vi "Dialog Window YN.vi"(6 "Front Panel Window:Panel Bounds":T2, 7 "Üzenet be":string, 8 "Error In":errorcluster, 10 "Message":T1, 11 "Message Queue":refnum<queue>) -> (0 "Error Out":errorcluster)   [LabVIEW 2014]
uses:
  <vilib>/Utility/miscctls.llb/LVRectTypeDef.ctl
  Message.ctl
  support/Message Queue/Message Cluster.ctl
  Teszt/Teszt.ctl
  Teszt/Command.ctl
  support/Message Queue/Enqueue Message (Single).vi
  support/Message Queue/Message Queue.lvlib
panel:
  in  "Nem":bool
  out "Üzenet":string
  in  "Igen":bool
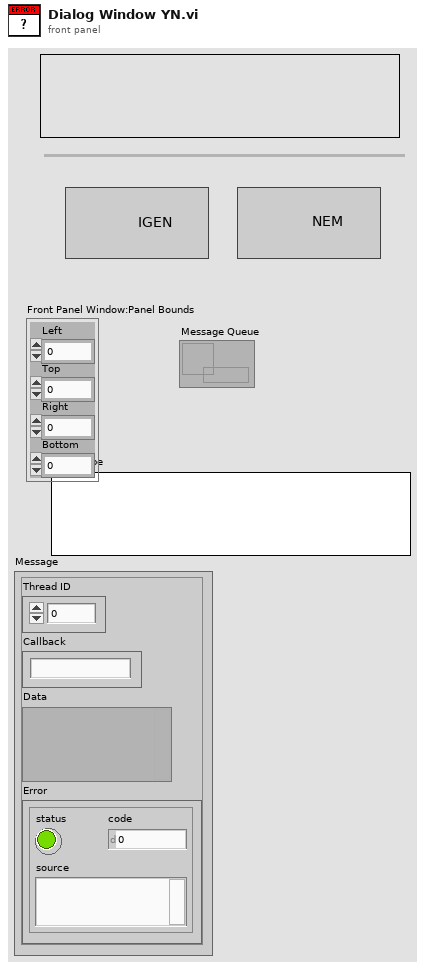
[diagram p1: front panel]
types:
  T1 = typedef "Message.ctl" = cluster{"Thread ID":u16, "Callback":string, "Data":variant, "Error":errorcluster}
  T2 = typedef "LVRectTypeDef.ctl" = cluster{"Left":i16, "Top":i16, "Right":i16, "Bottom":i16}
  T3 = typedef "Teszt.ctl" = cluster{"Thread ID":dbl, "Mérésszám":string, "Mérés/Utasítás":string, "Command":T4, "Min":string, "Max":string, "Aktív?":bool, "Log?":bool, "Kiértékelés":bool, "Etalon 1 exp":bool, "Etalon 2 exp":bool, "Etalon 3 exp":bool, "Etalon 4 exp":bool, "Etalon 5 exp":bool}
  T4 = typedef "Command.ctl" = cluster{"Parancs":string, "Paraméter 1":string, "Paraméter 2":string, "Paraméter 3":string, "Paraméter 4":string, "Paraméter 5":string, "Eredmény":string}
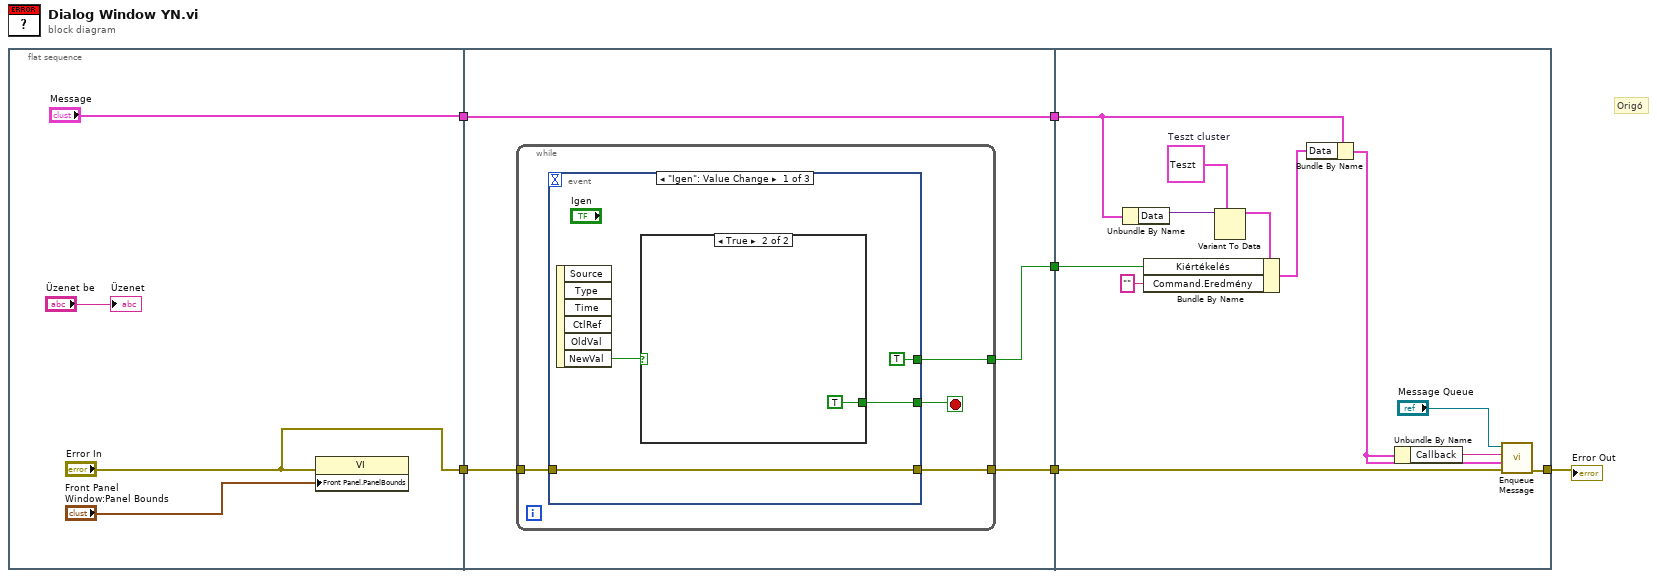
[diagram p0: block diagram]
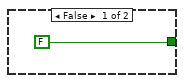
[diagram p2: hidden frame]
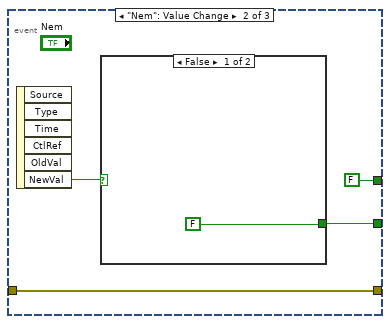
[diagram p3: hidden frame]
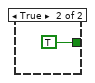
[diagram p4: hidden frame]
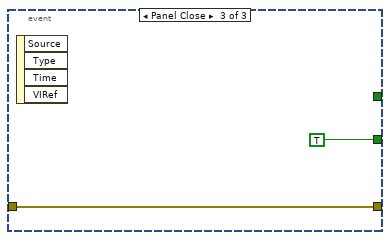
[diagram p5: hidden frame]
diagram:
  # "Origó"
  n1 = flat-sequence {
    tunnel: ["Error In"] -> w5
    tunnel: ["Message"] -> w3
    tunnel: w5 -> [w14]
    tunnel: [w13] -> w4
    tunnel: w3 -> [w12]
    tunnel: [w12] -> w2
    tunnel: [w11] -> w1
    tunnel: [w43] -> w6
    tunnel: w4 -> [w44]
    tunnel: w2 -> [w33]
    tunnel: w1 -> [w34]
    frame #0 {
      n2 = property on="Property Node" class="VI"(error in="Error In", "Front Panel.PanelBounds"="Front Panel Window:Panel Bounds") -> ()  [unwired: 1 in, 2 out]
      "Üzenet" <- "Üzenet be"
    }
    frame #1 {
      n3 = while {
        tunnel: w14 -> [w18]
        tunnel: [w17] -> w13
        tunnel: [w15] -> w11
        stop <- w16 stop-if-true
        n4 = event shown="[0] \"Igen\": Value Change" {
          selector: _ -> [_ _ _]
          dyn-events: _ -> [_ _ _]
          timeout: _ -> [_ _ _]
          tunnel: [w22 w28 w32] -> w17
          tunnel: w18 -> [w22 w28 w32]
          tunnel: [w20 w26 TRUE] -> w16
          tunnel: [TRUE FALSE _] -> w15
          event "Igen": Value Change {
            n5 = event-data() -> ("NewVal"=w21:bool)  [unwired: 1 in, 5 out]
            n6 = case shown="True" w21 {
              tunnel: [FALSE TRUE] -> w20
              frame False {
              }
              frame True {
              }
            }
          }
          event "Nem": Value Change {
            n7 = event-data() -> ("NewVal"=w27:bool)  [unwired: 1 in, 5 out]
            n8 = case shown="False" w27 {
              tunnel: [FALSE TRUE] -> w26
              frame False {
              }
              frame True {
              }
            }
          }
          event Panel Close {
            n9 = event-data() -> ()  [unwired: 1 in, 4 out]
          }
        }
      }
    }
    frame #2 {
      w37 = T3 {"Thread ID"=0.0, "Mérésszám"="", "Mérés/Utasítás"="", "Command"={"Parancs"="", "Paraméter 1"="", "Paraméter 2"="", "Paraméter 3"="", "Paraméter 4"="", "Paraméter 5"="", "Eredmény"=""}, "Min"="", "Max"="", "Aktív?"=FALSE, "Log?"=FALSE, "Kiértékelés"=FALSE, "Etalon 1 exp"=FALSE, "Etalon 2 exp"=FALSE, "Etalon 3 exp"=FALSE, "Etalon 4 exp"=FALSE, "Etalon 5 exp"=FALSE}  # Teszt cluster
      n10 = Unbundle By Name(w33) -> ("Data"=w36:variant)
      n11 = Variant To Data(type=w37, Variant=w36) -> (data=w39:T3)  [unwired: 1 in, 1 out]
      n12 = Bundle By Name(cluster=w39, "Kiértékelés"=w34, "Command.Eredmény"="") -> (w40:T3)
      n13 = Bundle By Name(cluster=w33, "Data"=w40) -> (w35:T1)
      n14 = Unbundle By Name(w35) -> ("Callback"=w41:string)
      n15 = call-poly "Enqueue Message.vi"("error in (no error)"=w44, "Message Data"=w35, "Message"=w41, "Message Queue"="Message Queue") -> ("error out"=w43:errorcluster)  [unwired: 6 in, 1 out]
    }
  }
  "Error Out" <- w6
